vi "XY Graph Smoothen Plot (Cubic Spline).vi"(6 "Tail only (F)":bool, 8 "error in (no error)":errorcluster, 9 "Replace Plot (T)?":bool=TRUE, 10 "balance parameter (-1: auto)":dbl=-1.0, 11 "Selected Plot Info":T1={"Multiplot XY Graph"=refnum, "Mouse Coordinates"={"Horizontal"=0, "Vertical"=0}, "Plot Index"=-1}) -> (0 "Error Out":errorcluster, 1 "Smooth Plot Message":string, 3 "Smoothed Plot":cluster{"X Array":dbl[], "Y Array":dbl[]})   [LabVIEW 2021, in "XY Graph Add-Ons.lvlib"]
uses:
  XY Graph Add-Ons.lvlib
  XY Graph Selected Plot Info.ctl
  XY Graph Refnum.ctl
  <vilib>/Utility/miscctls.llb/LVPoint32TypeDef.ctl
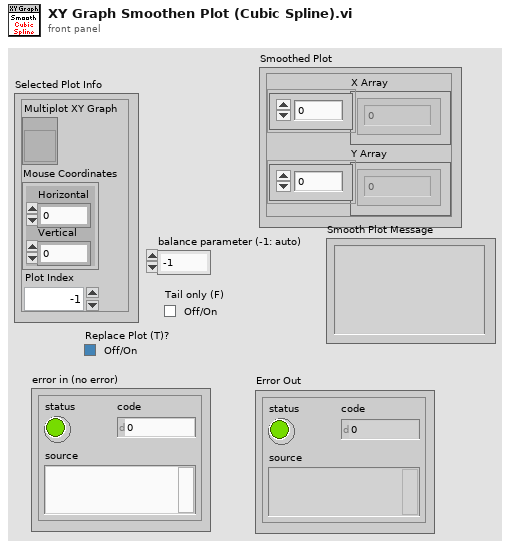
[diagram p1: front panel]
types:
  T1 = typedef "XY Graph Add-Ons.lvlib/XY Graph Selected Plot Info.ctl" = cluster{"Multiplot XY Graph":T2, "Mouse Coordinates":T3, "Plot Index":i32}
  T2 = typedef "XY Graph Add-Ons.lvlib/XY Graph Refnum.ctl" = refnum<vi>
  T3 = typedef "LVPoint32TypeDef.ctl" = cluster{"Horizontal":i32, "Vertical":i32}
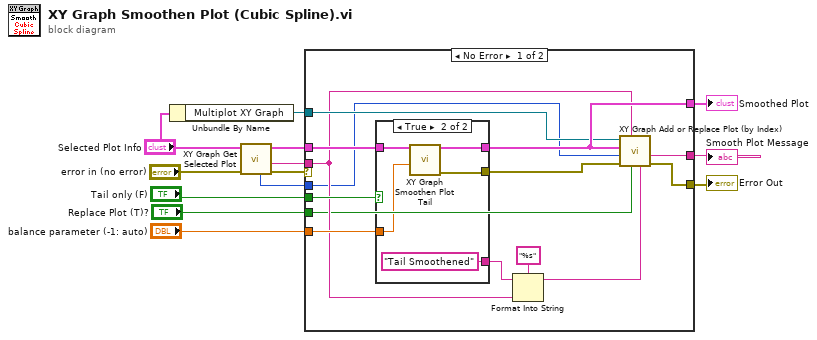
[diagram p0: block diagram]
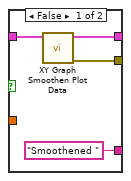
[diagram p2: hidden frame]
diagram:
  n1 = Unbundle By Name("Selected Plot Info") -> ("Multiplot XY Graph"=w3:T2)
  n2 = call "XY Graph Get Selected Plot.vi"("error in (no error)"="error in (no error)", "Selected Plot Info"="Selected Plot Info") -> ("error out"=w4:errorcluster, "Plot Name"=w5:string, "Plot"=w6:cluster{"X Array":dbl[], "Y Array":dbl[]}, "Plot Index in (dup)"=w7:i32)  [unwired: 4 in, 2 out]
  n3 = case shown="No Error" w4 {
    selector: w4 -> [_ w37]
    tunnel: [w22 _] -> w13
    tunnel: w5 -> [w19 _]
    tunnel: w7 -> [w18 _]
    tunnel: [w16 w37] -> w12
    tunnel: "Tail only (F)" -> [w26 _]
    tunnel: "balance parameter (-1: auto)" -> [w24 _]
    tunnel: w6 -> [w23 _]
    tunnel: w3 -> [w21 _]
    tunnel: [w15 _] -> w2
    tunnel: "Replace Plot (T)?" -> [w14 _]
    frame No Error {
      n4 = case shown="True" w26 {
        tunnel: w23 -> [w31 w36]
        tunnel: [w30 w35] -> w22
        tunnel: [w29 w34] -> w17
        tunnel: ["Smoothened " ("initial string") "Tail Smoothened" ("initial string")] -> w25
        tunnel: w24 -> [_ w32]
        frame False {
          n5 = call "XY Graph Smoothen Plot Data.vi"("Plot"=w31) -> ("error out"=w29:errorcluster, "Cubic Splined Plot"=w30:cluster{"X Array":dbl[], "Y Array":dbl[]})  [unwired: 9 in]
        }
        frame True {
          n6 = call "XY Graph Smoothen Plot Tail.vi"("balance parameter (-1: auto)"=w32, "Plot in"=w36) -> ("error out"=w34:errorcluster, "Plot out"=w35:cluster{"t Array":dbl[], "Y Array":dbl[]})  [unwired: 8 in]
        }
      }
      n7 = Format Into String(format string="%s", initial string=w25, w19) -> (resulting string=w20:string)  [unwired: 1 in, 1 out]
      n8 = call "XY Graph Add or Replace Plot (by Index).vi"("New Plot Name"=w20, "Replace Plot (T)?"=w14, "Original Plot Name"=w19, "error in (no error)"=w17, "Plot Index"=w18, "Plot in"=w22, "XYGraph in"=w21) -> ("error out"=w16:errorcluster, "Message"=w15:string)  [unwired: 3 in]
    }
    frame Error {
    }
  }
  "Error Out" <- w12
  "Smoothed Plot" <- w13
  "Smooth Plot Message" <- w2
